vi "3.1.vi"() -> ()   [LabVIEW 2017]
panel:
  out "余弦":dbl
  out "正弦":dbl
  in  "输入":dbl
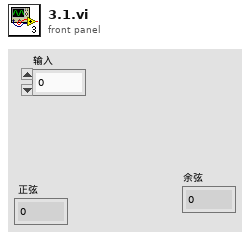
[diagram p1: front panel]
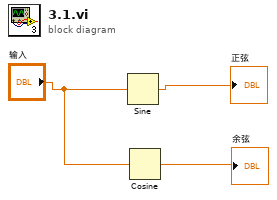
[diagram p0: block diagram]
diagram:
  n1 = Sine(x="输入") -> (sin(x)=→"正弦":dbl)
  n2 = Cosine(x="输入") -> (cos(x)=→"余弦":dbl)
